vi "OPC-UA-Item-Browser.vi"() -> ()   [LabVIEW 2015]
uses:
  <vilib>/OPCUA/NI OPC UA Client.lvlib
  <vilib>/OPCUA/NI OPC UA Utility.lvlib
panel:
  in  "server endpoint URL":string="opc.tcp://stfopc01.gsi.de:48010"
  in  "security policy":T1
  out "status":u32(ring) items=["Good"=0, "Bad_AttributeIdInvalid"=2153906176, "Bad_BrowseDirectionInvalid"=2152529920, "Bad_BrowseNameInvalid"=2153775104, "Bad_ContentFilterInvalid"=2152202240, "Bad_ContinuationPointInvalid"=2152333312, "Bad_DataEncodingInvalid"=2151153664, "Bad_DataEncodingUnsupported"=2151219200, "Bad_EventFilterInvalid"=2152136704, "Bad_FilterNotAllowed"=2152005632, "Bad_FilterOperandInvalid"=2160132096, "Bad_HistoryOperationInvalid"=2154889216, "Bad_HistoryOperationUnsupported"=2154954752, "Bad_IndexRangeInvalid"=2151022592, "Bad_IndexRangeNoData"=2151088128, "Bad_MonitoredItemFilterInvalid"=2151874560, "Bad_MonitoredItemFilterUnsupported"=2151940096, "Bad_MonitoredItemIdInvalid"=2151809024, "Bad_MonitoringModeInvalid"=2151743488, "Bad_NoCommunication"=2150694912, "Bad_NoContinuationPoints"=2152398848, "Bad_NodeClassInvalid"=2153709568, "Bad_NodeIdInvalid"=2150825984, "Bad_NodeIdUnknown"=2150891520, "Bad_NoDeleteRights"=2154364928, "Bad_NodeNotInView"=2152595456, "Bad_NotFound"=2151546880, "Bad_NotImplemented"=2151677952, "Bad_NotReadable"=2151284736, "Bad_NotSupported"=2151481344, "Bad_NotWritable"=2151350272, "Bad_ObjectDeleted"=2151612416, "Bad_OutOfRange"=2151415808, "Bad_ReferenceTypeIdInvalid"=2152464384, "Bad_SourceNodeIdInvalid"=2154037248, "Bad_StructureMissing"=2152071168, "Bad_TargetNodeIdInvalid"=2154102784, "Bad_TypeDefinitionInvalid"=2153971712, "Bad_TypeMismatch"=2155085824, "Bad_WaitingForInitialData"=2150760448]
  in  "node type":enum32{"Other", "Folder", "Item/Property"}(ring)=enum."Item/Property"
  out "sorted array":T2(array[cluster])
  out "size(s)":i32
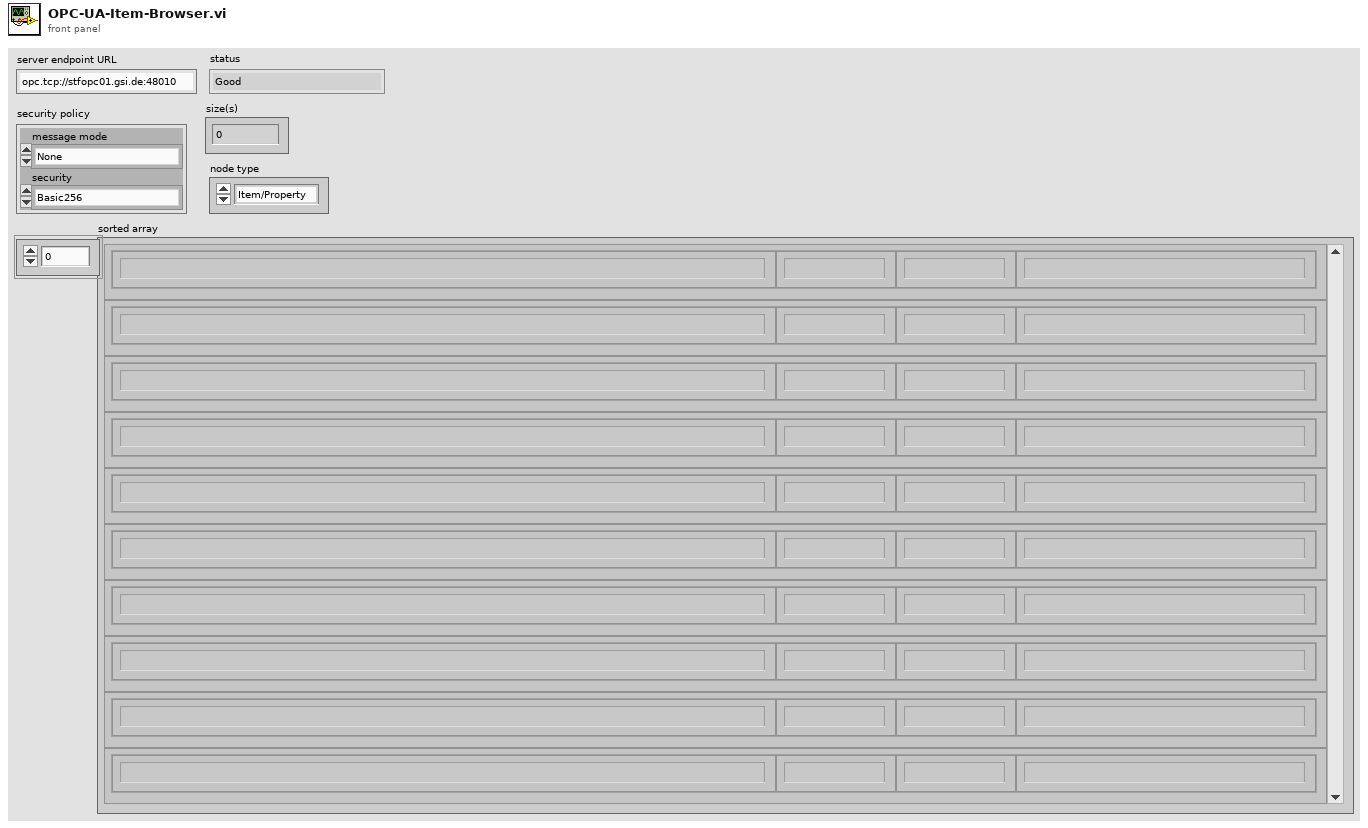
[diagram p1: front panel]
types:
  T1 = cluster{"message mode":enum16{"None", "Sign", "Sign and Encrypt"}, "security":enum16{"Basic256", "Basic128Rsa15"}}
  T2 = cluster{"node name":string, "String":string, "String":string, "node path":string}[]
  T3 = cluster{"node path":string, string, string, "node name":string}[]
  T4 = cluster{"node path":string, "node name":string, "node type":enum32{"Other", "Folder", "Item/Property"}}[]
  T5 = cluster{"status":u32, "browse result":cluster{"node path":string, "node name":string, "node type":enum32{"Other", "Folder", "Item/Property"}}[], i32}
  T6 = cluster{"node path":string, string, string, "node name":string}
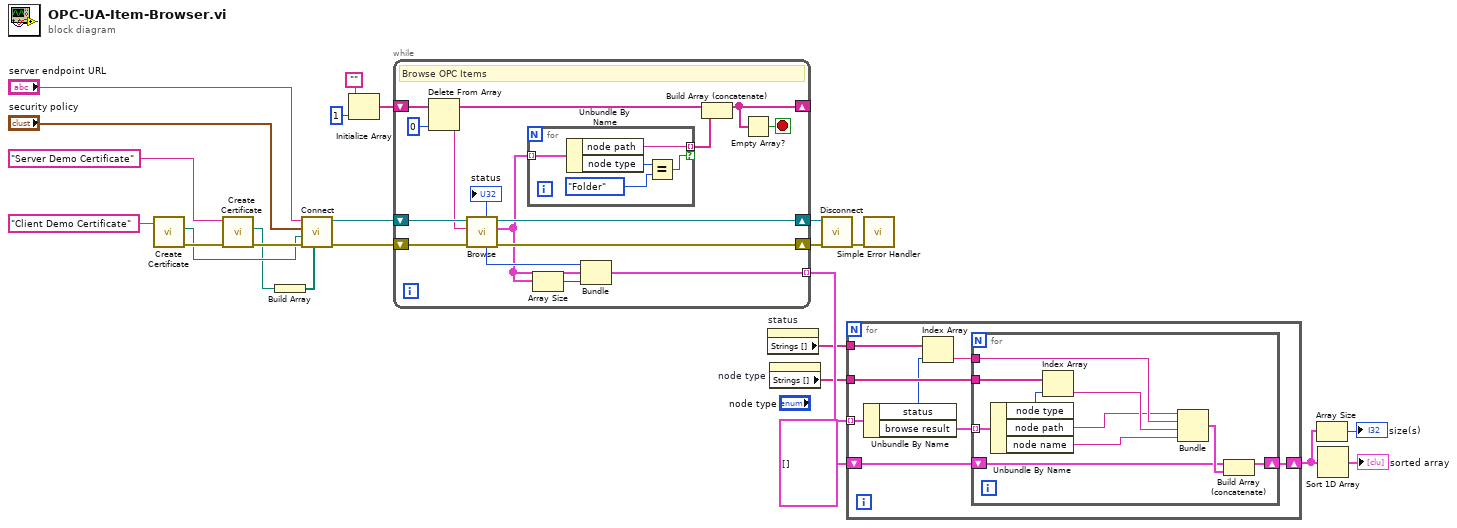
[diagram p0: block diagram]
diagram:
  n1 = call <vilib>:"Create Certificate.vi"("certificate name in"="Client Demo Certificate") -> ("error out"=w22:errorcluster, "certificate path"=w17:path)  [unwired: 7 in, 2 out]
  n2 = call <vilib>:"Create Certificate.vi"("error in (no error)"=w22, "certificate name in"="Server Demo Certificate") -> ("error out"=w21:errorcluster, "certificate path"=w16:path)  [unwired: 6 in, 2 out]
  n3 = Build Array(w16) -> (w19:path[])
  n4 = call <vilib>:"Connect.vi"("trusted server certificates"=w19, "error in (no error)"=w21, "client certificate file"=w17, "security policy"="security policy", "server endpoint URL"="server endpoint URL") -> ("error out"=w11:errorcluster, "OPC UA client refnum out"=w12:refnum<k21>)  [unwired: 4 in, 1 out]
  n5 = Initialize Array("", 1 ("dimension size")) -> (w8:string[])
  n6 = while {
    shift-right: [w36] -> w13
    shift-left: w11 -> [w39]
    shift-right: [w37] -> w14
    shift-left: w12 -> [w38]
    shift-right: [w29] -> _
    shift-left: w8 -> [w34]
    tunnel: [w27] -> w7 mode=indexing
    stop <- w30 stop-if-true
    # "Browse OPC Items"
    n7 = Delete From Array(array=w34, index=0) -> (deleted portion=w32:string, array with subset deleted=w33:string[])  [unwired: 1 in]
    n8 = call <vilib>:"Browse.vi"("error in (no error)"=w39, "node path"=w32, "OPC UA client refnum in"=w38) -> ("error out"=w36:errorcluster, "status"=w28:u32, "browse result"=w26:T4, "OPC UA client refnum out"=w37:refnum<k21>)  [unwired: 5 in]
    "status" <- w28
    n9 = for {
      tunnel: w26 -> [w44] mode=indexing
      tunnel: [w43] -> w35 mode=indexing if=w42
      n10 = Unbundle By Name(w44) -> ("node path"=w43:string, "node type"=w41:enum32{"Other", "Folder", "Item/Property"})
      n11 = Equal?(x=w41, y=enum32{"Other", "Folder", "Item/Property"}."Folder" ("node type")) -> (x = y?=w42:bool)
    }
    n12 = Array Size(array=w26) -> (size(s)=w25:i32)
    n13 = Bundle("status"=w28, "browse result"=w26, w25) -> (w27:T5)  [unwired: 1 in]
    n14 = Build Array (concatenate)(w33, w35) -> (w29:string[])
    n15 = Empty Array?(array=w29) -> (empty?=w30:bool)
  }
  n16 = property on="status" class="Ring (strict)"() -> ("Strings []"=w5:string[])  [unwired: 2 in, 2 out]
  n17 = property on="node type" class="Enum (strict)"() -> ("Strings []"=w6:string[])  [unwired: 2 in, 2 out]
  n18 = call <vilib>:"Disconnect.vi"("error in (no error)"=w13, "OPC UA client refnum in"=w14) -> ("error out"=w15:errorcluster)  [unwired: 9 in]
  n19 = for {
    tunnel: w7 -> [w52] mode=indexing
    tunnel: w6 -> [w50]
    tunnel: w5 -> [w48]
    shift-right: [w46] -> w3
    shift-left: T3 [] -> [w45]
    n20 = Unbundle By Name(w52) -> ("status"=w49:u32, "browse result"=w51:T4)
    n21 = Index Array(array=w48, index=w49) -> (element=w47:string)
    n22 = for {
      tunnel: w51 -> [w62] mode=indexing
      tunnel: w50 -> [w61]
      tunnel: w47 -> [w60]
      shift-right: [w56] -> w46
      shift-left: w45 -> [w55]
      n23 = Unbundle By Name(w62) -> ("node type"=w59:enum32{"Other", "Folder", "Item/Property"}, "node path"=w53:string, "node name"=w54:string)
      n24 = Index Array(array=w61, index=w59) -> (element=w58:string)
      n25 = Bundle("node path"=w53, w60, w58, "node name"=w54) -> (w57:T6)  [unwired: 1 in]
      n26 = Build Array (concatenate)(w55, w57) -> (w56:T3)
    }
  }
  n27 = call <vilib>:"Simple Error Handler.vi"("error in (no error)"=w15) -> ()  [unwired: 4 in, 5 out]
  n28 = Array Size(array=w3) -> (size(s)=→"size(s)":i32)
  n29 = Sort 1D Array(array=w3) -> (sorted array=→"sorted array":T3)
